vi "Remote Calibration Variable.vi"() -> ()   [LabVIEW 2014]
uses:
  Remote Calibration Typedef.ctl
panel:
  in  "Remote Calibration Parameters":T1={"Rear BP Scaling Factor"=1250.0, "Front BP Scaling Factor"=1250.0, "Rear BP Offset (V)"=0.4820899963378906, "Front BP Offset"=0.4808177947998047, "Throttle 2 Max"=3.89990234375, "Throttle 2 Min"=2.090087890625, "Throttle 1 Max"=0.6298828125, "Throttle 1 Min"=2.4599609375, "MC Update Period (ms)"=40, "Regen Mult."=0.0, "Zero Torque %"=0.0, "Torque Mult."=120.0, "Activation Brake Pressure"=-1.0}
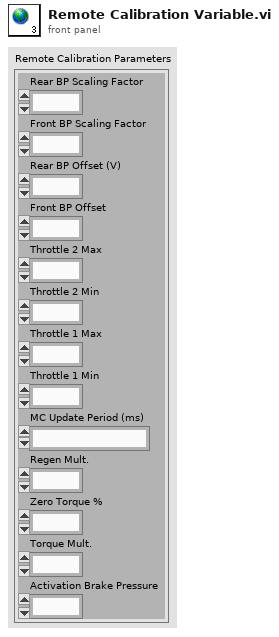
[diagram p1: front panel]
types:
  T1 = typedef "Remote Calibration Typedef.ctl" = cluster{"Rear BP Scaling Factor":fxp<+,11,11>, "Front BP Scaling Factor":fxp<+,11,11>, "Rear BP Offset (V)":fxp<+/-,26,5>, "Front BP Offset":fxp<+/-,26,5>, "Throttle 2 Max":fxp<+,16,4>, "Throttle 2 Min":fxp<+,16,4>, "Throttle 1 Max":fxp<+,16,4>, "Throttle 1 Min":fxp<+,16,4>, "MC Update Period (ms)":u32, "Regen Mult.":dbl, "Zero Torque %":dbl, "Torque Mult.":dbl, "Activation Brake Pressure":dbl}
diagram:
